vi "BuildDataLogConfiguration.vi"(8 "error in (no error)":errorcluster, 9 "Channel Paths":string[](array[string]), 10 "Rate [Hz]":dbl=100.0, 11 "Log File Path (temporary file)":path) -> (0 "error out":errorcluster, 3 "Data Log File Configuration":T1)   [LabVIEW 2015, in "VeriStandTestUtilities.lvlib"]
uses:
  VeriStandTestUtilities/VeriStandTestUtilities.lvlib
  <vilib>/NI Veristand/Execution/Workspace/LogFileConfiguration.ctl
  <vilib>/NI Veristand/Execution/Workspace/LogFileTriggerConfiguration.ctl
  <vilib>/NI Veristand/Execution/Workspace/LogFileTriggerType.ctl
  <vilib>/NI Veristand/Execution/Workspace/LogProperty.ctl
  <vilib>/NI Veristand/Execution/Workspace/LogChannelConfiguration.ctl
  <vilib>/NI VeriStand/Execution/Workspace/NI_VS Workspace ExecutionAPI.lvlib
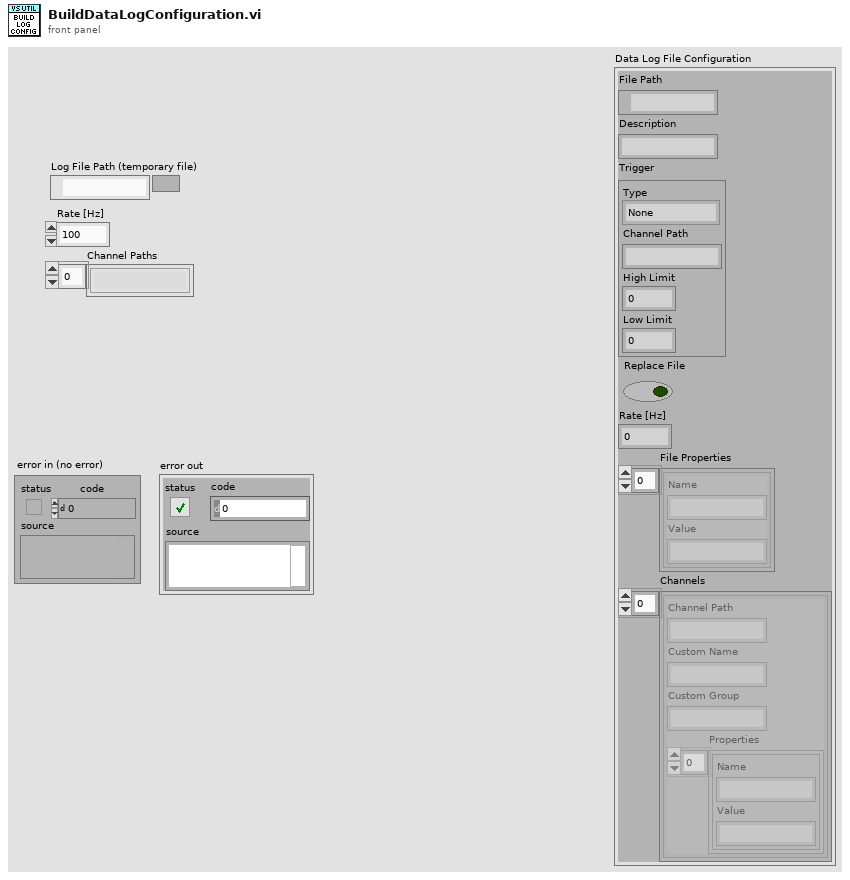
[diagram p1: front panel]
types:
  T1 = typedef "NI_VS Workspace ExecutionAPI.lvlib/LogFileConfiguration.ctl" = cluster{"File Path":path, "Description":string, "Trigger":T2, "Replace File":bool, "Rate [Hz]":dbl, "File Properties":T4[], "Channels":T5[]}
  T2 = typedef "NI_VS Workspace ExecutionAPI.lvlib/LogFileTriggerConfiguration.ctl" = cluster{"Type":T3, "Channel Path":string, "High Limit":dbl, "Low Limit":dbl}
  T3 = typedef "NI_VS Workspace ExecutionAPI.lvlib/LogFileTriggerType.ctl" = enum16{"None", "In Limits", "Out of Limits"}
  T4 = typedef "NI_VS Workspace ExecutionAPI.lvlib/LogProperty.ctl" = cluster{"Name":string, "Value":string}
  T5 = typedef "NI_VS Workspace ExecutionAPI.lvlib/LogChannelConfiguration.ctl" = cluster{"Channel Path":string, "Custom Name":string, "Custom Group":string, "Properties":T4[]}
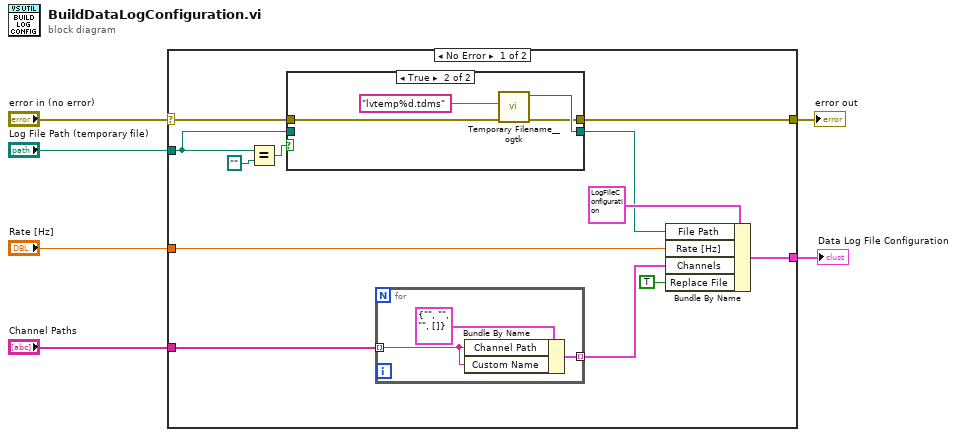
[diagram p0: block diagram]
diagram:
  n1 = case shown="No Error" "error in (no error)" {
    selector: "error in (no error)" -> [w12 w28]
    tunnel: [w11 w28] -> w5
    tunnel: "Log File Path (temporary file)" -> [w10 _]
    tunnel: "Channel Paths" -> [w9 _]
    tunnel: "Rate [Hz]" -> [w8 _]
    tunnel: [w7 _] -> w1
    frame No Error {
      n2 = Equal?(x=w10, y=path "") -> (x = y?=w15:bool)
      n3 = case shown="True" w15 {
        tunnel: [w20 w23] -> w14
        tunnel: w10 -> [w20 _]
        tunnel: w12 -> [w19 w22]
        tunnel: [w19 w21] -> w11
        frame False {
        }
        frame True {
          n4 = call <userlib>:"Temporary Filename__ogtk.vi"("error in (no error)"=w22, "pattern (lvtemp%d.tmp)"="lvtemp%d.tdms") -> ("error out"=w21:errorcluster, "file in tmp dir"=w23:path)  [unwired: 4 in]
        }
      }
      n5 = for {
        tunnel: w9 -> [w25] mode=indexing
        tunnel: [w27] -> w17 mode=indexing
        n6 = Bundle By Name(cluster=T5 {"Channel Path"="", "Custom Name"="", "Custom Group"="", "Properties"=[]} ("LogChannelInfo"), "Channel Path"=w25, "Custom Name"=w25) -> (w27:T5)
      }
      n7 = Bundle By Name(cluster=T1 {"File Path"=path "", "Description"="", "Trigger"={"Type"=enum."None", "Channel Path"="", "High Limit"=0.0, "Low Limit"=0.0}, "Replace File"=FALSE, "Rate [Hz]"=1.0, "File Properties"=[], "Channels"=[]} ("Data Log File Configuration"), "File Path"=w14, "Rate [Hz]"=w8, "Channels"=w17, "Replace File"=TRUE) -> (w7:T1)
    }
    frame Error {
    }
  }
  "error out" <- w5
  "Data Log File Configuration" <- w1
